vi "BK9120 Ramp Control.vi"(8 "Error In":errorcluster, 10 "Current":refnum<vi>, 11 "B&K In":refnum<class "B&K Precision 9120 series.lvclass">) -> (0 "Error Out":errorcluster, 3 "B&K Out":refnum<class "B&K Precision 9120 series.lvclass">)   [LabVIEW 2014]
uses:
  BK9120/B&K Precision 9120 series.lvclass
panel:
  out "millisecond timer value":u32
  out "Time":u32
  out "Ramp up interval":u32
  out "Ramp On":bool
  out "Current Setpoint":dbl format="%p A"
  in  "Exit":bool
  in  "Ramp up rate":dbl=0.005 min=-1.0 max=1.0 step=0.0010000000474974513 format="%#_p A/min"
  in  "Stop Ramp":bool
  in  "Start Ramp":bool
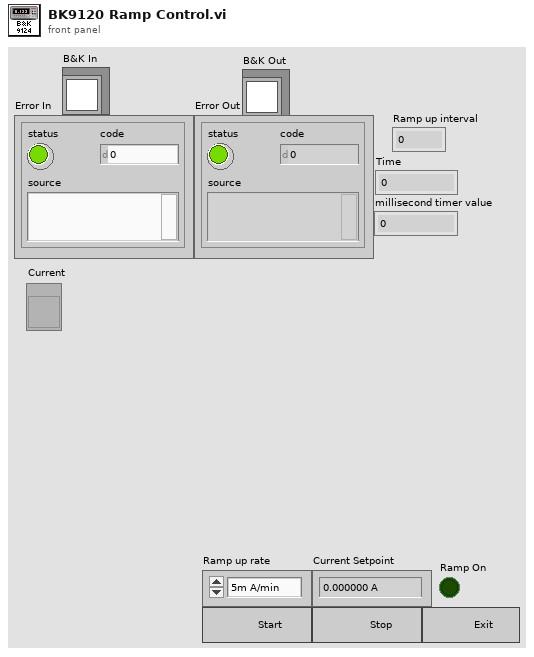
[diagram p1: front panel]
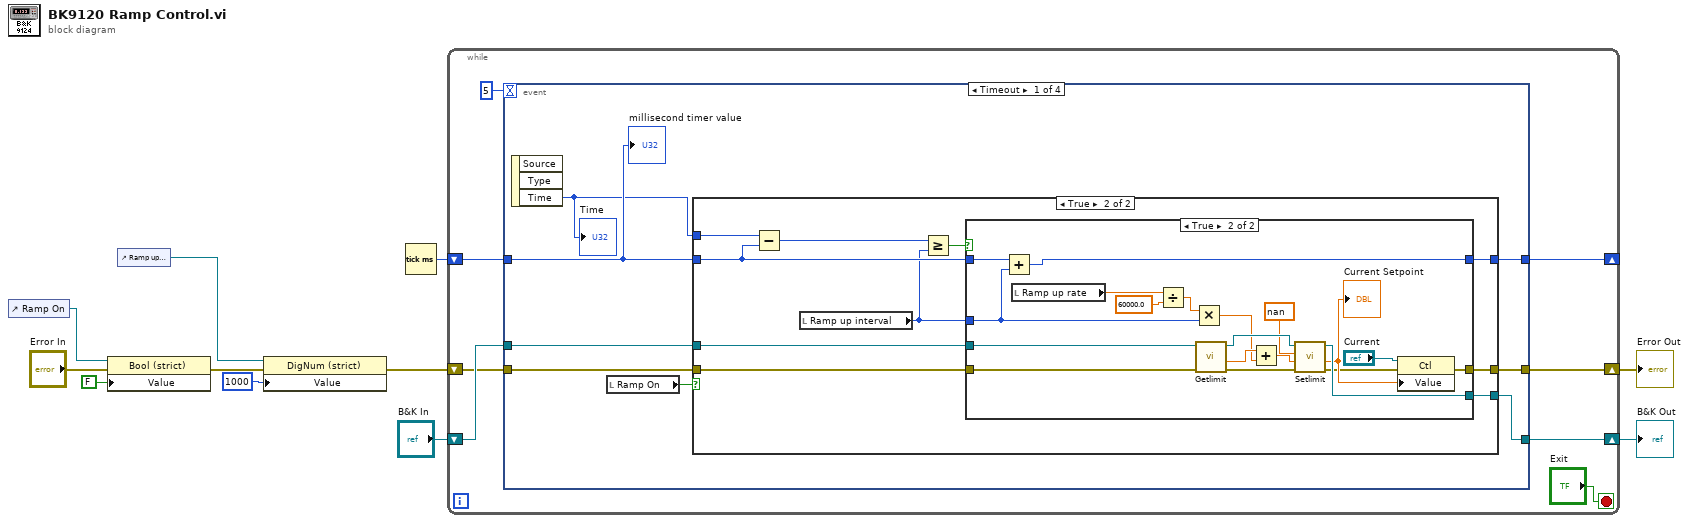
[diagram p0: block diagram]
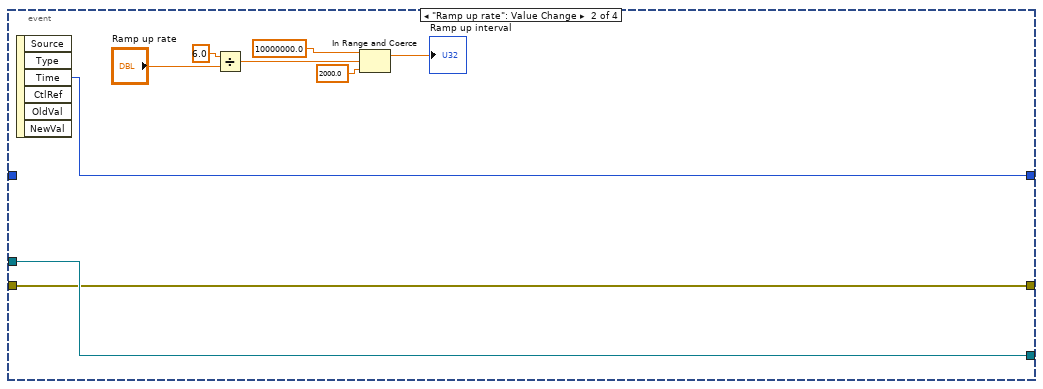
[diagram p4: hidden frame]
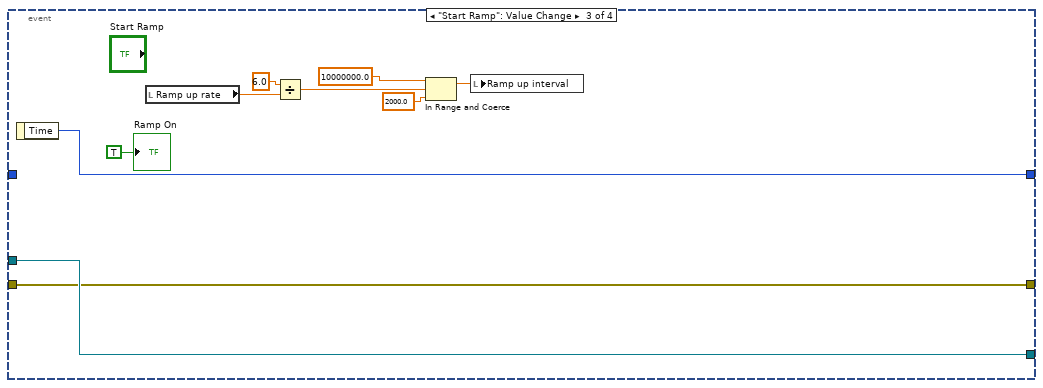
[diagram p5: hidden frame]
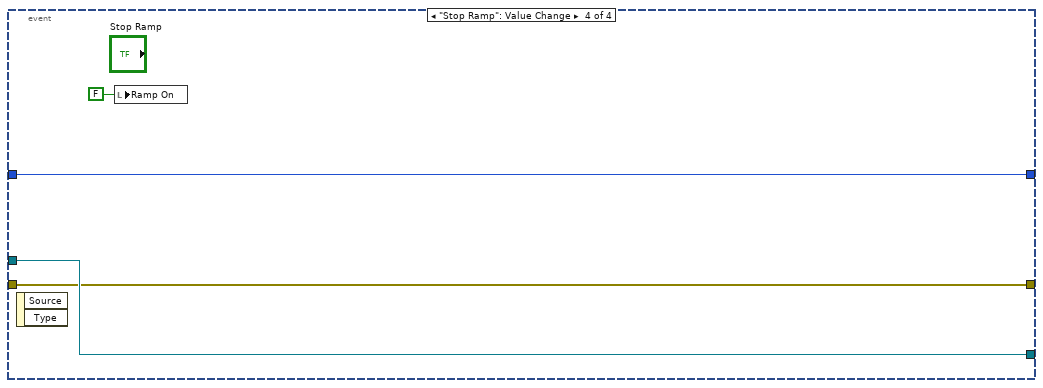
[diagram p6: hidden frame]
diagram:
  n1 = control-ref of="Ramp On"() -> (w11:refnum<vi>)
  n2 = property class="Bool (strict)"(reference=w11, error in="Error In", "Value"=FALSE) -> (error out=w8:errorcluster)  [unwired: 1 out]
  n3 = control-ref of="Ramp up interval"() -> (w6:refnum<vi>)
  n4 = property class="DigNum (strict)"(reference=w6, error in=w8, "Value"=i64 1000 ("Period")) -> (error out=w7:errorcluster)  [unwired: 1 out]
  n5 = Tick Count (ms)() -> (millisecond timer value=w1:u32)
  n6 = while {
    shift-right: [w14] -> w4
    shift-left: w7 -> [w15]
    shift-right: [w16] -> w2
    shift-left: "B&K In" -> [w17]
    shift-right: [w12] -> _
    shift-left: w1 -> [w13]
    stop <- "Exit" stop-if-true
    n7 = event shown="[0] Timeout" {
      selector: _ -> [_ _ _ _]
      dyn-events: _ -> [_ _ _ _]
      timeout: 5 -> [_ _ _ _]
      tunnel: w17 -> [w26 w71 w80 w84]
      tunnel: [w24 w71 w80 w84] -> w16
      tunnel: w15 -> [w25 w70 w79 w83]
      tunnel: [w23 w70 w79 w83] -> w14
      tunnel: w13 -> [w22 _ _ w82]
      tunnel: [w21 w63 w72 w82] -> w12
      event Timeout {
        n8 = event-data() -> ("Time"=w20:u32)  [unwired: 1 in, 2 out]
        "Time" <- w20
        n9 = local read "Ramp On"() -> (w27:bool)
        n10 = case shown="True" w27 {
          tunnel: w26 -> [w30 w40]
          tunnel: [w30 w38] -> w24
          tunnel: w25 -> [w29 w39]
          tunnel: [w29 w37] -> w23
          tunnel: w22 -> [w28 w35]
          tunnel: [w28 w36] -> w21
          tunnel: w20 -> [_ w31]
          frame False {
          }
          frame True {
            n11 = Subtract(x=w31, y=w35) -> (x-y=w34:u32)
            n12 = local read "Ramp up interval"() -> (w33:u32)
            n13 = Greater Or Equal?(x=w34, y=w33) -> (x >= y?=w32:bool)
            n14 = case shown="True" w32 {
              tunnel: w40 -> [w41 w62]
              tunnel: w39 -> [w42 w61]
              tunnel: [w41 w59] -> w38
              tunnel: [w42 w45] -> w37
              tunnel: [w43 w49] -> w36
              tunnel: w33 -> [_ w50]
              tunnel: w35 -> [w43 w51]
              frame False {
              }
              frame True {
                n15 = Add(x=w51, y=w50) -> (x+y=w49:u32)
                n16 = local read "Ramp up rate"() -> (w52:dbl)
                n17 = Divide(x=w52, y=60000.0) -> (x/y=w54:dbl)
                n18 = Multiply(x=w54, y=w50) -> (x*y=w53:dbl)
                n19 = call "Getlimit.vi"("error in (no error)"=w61, "B&K Precision 9120 series in"=w62) -> ("error out"=w58:errorcluster, "Current read"=w57:dbl, "B&K Precision 9120 series out"=w60:refnum<class "B&K Precision 9120 series.lvclass">)  [unwired: 6 in, 1 out]
                n20 = Add(x=w57, y=w53) -> (x+y=w56:dbl)
                n21 = call "Setlimit.vi"("error in (no error)"=w58, "Current"=w56, "Voltage"=nan, "B&K Precision 9120 series in"=w60) -> ("error out"=w46:errorcluster, "Current read"=w47:dbl, "B&K Precision 9120 series out"=w59:refnum<class "B&K Precision 9120 series.lvclass">)  [unwired: 4 in, 1 out]
                "Current Setpoint" <- w47
                n22 = property class="Ctl"(reference="Current", error in=w46, "Value"=w47) -> (error out=w45:errorcluster)  [unwired: 1 out]
              }
            }
          }
        }
        "millisecond timer value" <- w22
      }
      event "Ramp up rate": Value Change {
        n23 = event-data() -> ("Time"=w63:u32)  [unwired: 1 in, 5 out]
        n24 = Divide(x=6.0 ("y"), y="Ramp up rate") -> (x/y=w64:dbl)
        n25 = In Range and Coerce(upper limit=10000000.0, x=w64, lower limit=2000.0) -> (coerced(x)=→"Ramp up interval":dbl)  [unwired: 1 out]
      }
      event "Start Ramp": Value Change {
        n26 = event-data() -> ("Time"=w72:u32)  [unwired: 1 in]
        n27 = local read "Ramp up rate"() -> (w74:dbl)
        n28 = Divide(x=6.0 ("y"), y=w74) -> (x/y=w73:dbl)
        n29 = In Range and Coerce(upper limit=10000000.0, x=w73, lower limit=2000.0) -> (coerced(x)=w76:dbl)  [unwired: 1 out]
        n30 = local write "Ramp up interval"(w76) -> ()
        "Ramp On" <- TRUE
      }
      event "Stop Ramp": Value Change {
        n31 = event-data() -> ()  [unwired: 1 in, 2 out]
        n32 = local write "Ramp On"(FALSE) -> ()
      }
    }
  }
  "B&K Out" <- w2
  "Error Out" <- w4
